vi "RT Driver VI.vi"(7 "Operation":T1, 11 "Device Reference in":T2 format="%.0x") -> (0 "Error Code":i32)   [LabVIEW 2019, in "FPGA Addon Engine.lvlib"]
uses:
  FPGA Addon Engine.lvlib
  <vilib>/rvi/interface/nirviCloseFPGA/nirviCloseFPGA.xnode
  <vilib>/FPGAPlugInAG/Dynamic/niLvFpga_Close_Dynamic.vi
  <vilib>/NI VeriStand/Custom Device API/Custom Device API.lvlib
  <vilib>/rvi/interface/nirviMethod/nirviMethod.xnode
  <vilib>/rvi/interface/nirviMethod/StockFPGA_InlinedMethodWaitForSingleIRQ.vi
  <vilib>/FPGAPlugInAG/Dynamic/niLvFpga_WaitOnIrq_Dynamic.vi
  <vilib>/FPGAPlugInAG/Dynamic/niLvFpga_AcknowledgeIrq_Dynamic.vi
  <vilib>/NI/NIVS Inline Async API/_VS Inline Async API/VS Inline Async API/VS Inline Async API.lvclass
  <vilib>/NI VeriStand/Custom Device Waveform API/Multiple Waveforms Write (DBL)/Multiple Waveforms Write (DBL).lvclass
  <vilib>/NI VeriStand/Custom Device Waveform API/Single Waveform Read (DBL)/Single Waveform Read (DBL).lvclass
  <vilib>/NI VeriStand/Custom Device API/Custom Device Item Ref.ctl
  <vilib>/NI VeriStand/Custom Device API/Hardware Interface Driver VI Operation.ctl
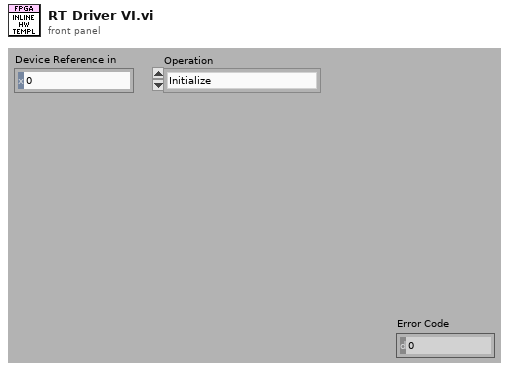
[diagram p1: front panel]
types:
  T1 = typedef "Custom Device API.lvlib/Hardware Interface Driver VI Operation.ctl" = enum16{"Initialize", "Start", "Read Data from HW", "Write Data to HW", "Close"}
  T2 = typedef "Custom Device API.lvlib/Custom Device Item Ref.ctl" = u64
  T3 = typedef "FPGA Addon Engine.lvlib/State Variables.ctl" = cluster{"FPGA Ref":refnum<k20>, "IncomingRegisters.Refs":T4[], "IncomingDMA.Refs":T7[], "OutgoingRegisters.Refs":T4[], "OutgoingDMA.Refs":T12[], "Compiled":T14}
  T4 = typedef "FPGA Addon Engine.lvlib/Register Settings.ctl" = cluster{"Data Type":T5, "U64":refnum<k20>, "U32":refnum<k20>, "U16":refnum<k20>, "U8":refnum<k20>, "I64":refnum<k20>, "I32":refnum<k20>, "I16":refnum<k20>, "I8":refnum<k20>, "SGL":refnum<k20>, "Bool":refnum<k20>, "Scalar Type":T6, "Index":i32, "Length":i32, "Analog PWM In":refnum<k20>, "Digital PWM In":refnum<k20>, "Digital PWM Out":refnum<k20>, "Analog PWM In Settings":refnum<k20>, "Digital PWM In Settings":refnum<k20>, "Sine Out":refnum<k20>, "FXP+/-24.5":refnum<k20>, "FXP+/-16.5":refnum<k20>, "FXP+/-32.8":refnum<k20>, "FXP+/-64.32":refnum<k20>, "FXP+/-16.7":refnum<k20>, "FXP+/-20.5":refnum<k20>, "FXP+/-27.5":refnum<k20>, "FXP+/-32.16":refnum<k20>, "FXP+16.3":refnum<k20>, "FXP+18.3":refnum<k20>, "Digital Static In":refnum<k20>, "Digital Static Out":refnum<k20>, "Digital Static In Settings":refnum<k20>, "Digital WSS Out":refnum<k20>, "Quad Encoder Settings":refnum<k20>, "Quad Encoder In":refnum<k20>}
  T5 = typedef "FPGA Addon Shared.lvlib/Data Type.ctl" = enum8{"<Null>", "I8", "I16", "I32", "I64", "U8", "U16", "U32", "U64", "SGL", "Boolean", "Analog PWM In Settings", "Analog PWM In", "Digital PWM In Settings", "Digital PWM In", "Digital PWM Out", "Sine Out", "FXP+/-24.5", "FXP+/-16.5", "FXP+/-32.8", "FXP+/-64.32", "FXP+/-16.7", "FXP+/-20.5", "FXP+/-27.5", "FXP+/-32.16", "FXP+16.3", "FXP+18.3", "Digital Static In", "Digital Static Out", "Digital Static In Settings", "Digital WSS Out", "Quad Encoder Settings", "Quad Encoder In", "Group"}
  T6 = typedef "FPGA Addon Shared.lvlib/Scalar Type.ctl" = enum16{"Standard", "Bitpacked"}
  T7 = typedef "FPGA Addon Engine.lvlib/DMA Input References.ctl" = cluster{"Addon Name":string, "Waveform Ref":refnum<class "Multiple Waveforms Write (DBL).lvclass">, "DMA Name":string, "DMA Settings":T8, "Refs":T11}
  T8 = typedef "FPGA Addon Shared.lvlib/DMA Settings.ctl" = cluster{"Number of Channels":u8, "Delacing Scheme":T9, "Update Rate":u32, "dt":dbl, "Mode":T10, "Number of Samples":u32, "DMA Host Buffer":u32}
  T9 = typedef "FPGA Addon Shared.lvlib/Delacing Scheme.ctl" = enum8{"Interleaved", "Bitpacked"}
  T10 = typedef "FPGA Addon Shared.lvlib/DMA Acquisition Mode.ctl" = enum8{"Continuous", "Triggered Finite"}
  T11 = typedef "FPGA Addon Engine.lvlib/DMA Input Refs.ctl" = cluster{"Data Type":T5, "DMA_SGL":refnum<k20>, "DMA_U64":refnum<k20>, "DMA_I64":refnum<k20>, "DMA_FXP+/-32.8":refnum<k20>, "DMA_FXP+/-64.32":refnum<k20>, "DMA_U32":refnum<k20>, "DMA_U16":refnum<k20>, "DMA_U8":refnum<k20>, "DMA_I32":refnum<k20>, "DMA_I16":refnum<k20>, "DMA_I8":refnum<k20>, "DMA_FXP+/-32.16":refnum<k20>}
  T12 = typedef "FPGA Addon Engine.lvlib/DMA Output References.ctl" = cluster{"Addon Name":string, "Waveforms":refnum<class "Single Waveform Read (DBL).lvclass">[], "DMA Name":string, "Refs":T13}
  T13 = typedef "FPGA Addon Engine.lvlib/DMA Output Refs.ctl" = cluster{"Data Type":T5, "DMA_SGL":refnum<k20>, "DMA_U64":refnum<k20>, "DMA_I64":refnum<k20>, "DMA_FXP+/-32.8":refnum<k20>, "DMA_FXP+/-64.32":refnum<k20>, "DMA_U32":refnum<k20>, "DMA_U16":refnum<k20>, "DMA_U8":refnum<k20>, "DMA_I32":refnum<k20>, "DMA_I16":refnum<k20>, "DMA_I8":refnum<k20>, "DMA_FXP+/-32.16":refnum<k20>}
  T14 = typedef "FPGA Addon Shared.lvlib/Compiled.Settings.ctl" = cluster{"Name":string, "IncomingRegisters.Settings":T15[], "IncomingRegisters.Refs":cluster{"Refs":T17[], "Values":dbl[]}, "OutgoingRegisters.Settings":T15[], "OutgoingRegisters.Refs":cluster{"Refs":T17[], "Values":dbl[]}, "Incoming.Size":i32, "Outgoing.Size":i32, "IncomingDMA.Settings":T19[], "OutgoingDMA.Settings":T19[], "FPGA.Settings":T21, "Target.Type":T22}
  T15 = typedef "FPGA Addon Shared.lvlib/Compiled.RegisterSettings.ctl" = cluster{"Scalar Type":T6, "Index":i32, "Length":i32, "Register":T16}
  T16 = typedef "FPGA Addon Shared.lvlib/Register Information.ctl" = cluster{"Name":string, "Data Type":T5, "Default Value":variant}
  T17 = typedef "Custom Device API.lvlib/Block Data Reference.ctl" = cluster{"Data Reference":T18, "Offset":u64, "Length":u64}
  T18 = typedef "Custom Device API.lvlib/Data Reference.ctl" = i32
  T19 = typedef "FPGA Addon Shared.lvlib/Compiled.DMASettings.ctl" = cluster{"Name":string, "Data Type":T5, "DMA.Settings":T8, "DMA.VSRefs":T20[]}
  T20 = typedef "Custom Device API.lvlib/Waveform Data Reference.ctl" = i32
  T21 = typedef "FPGA Addon Shared.lvlib/FPGA Settings.ctl" = cluster{"Bitfile path":path, "RIO Device Address":string, "Group":bool}
  T22 = typedef "Custom Device API.lvlib/Custom Device Target Type.ctl" = enum16{"PharLap", "VxWorks", "Windows", "Linux_32_ARM", "Linux_x64"}
  T23 = cluster{"Vars":T3, "Async?":bool, "Async":refnum<class "VS Inline Async API.lvclass">}
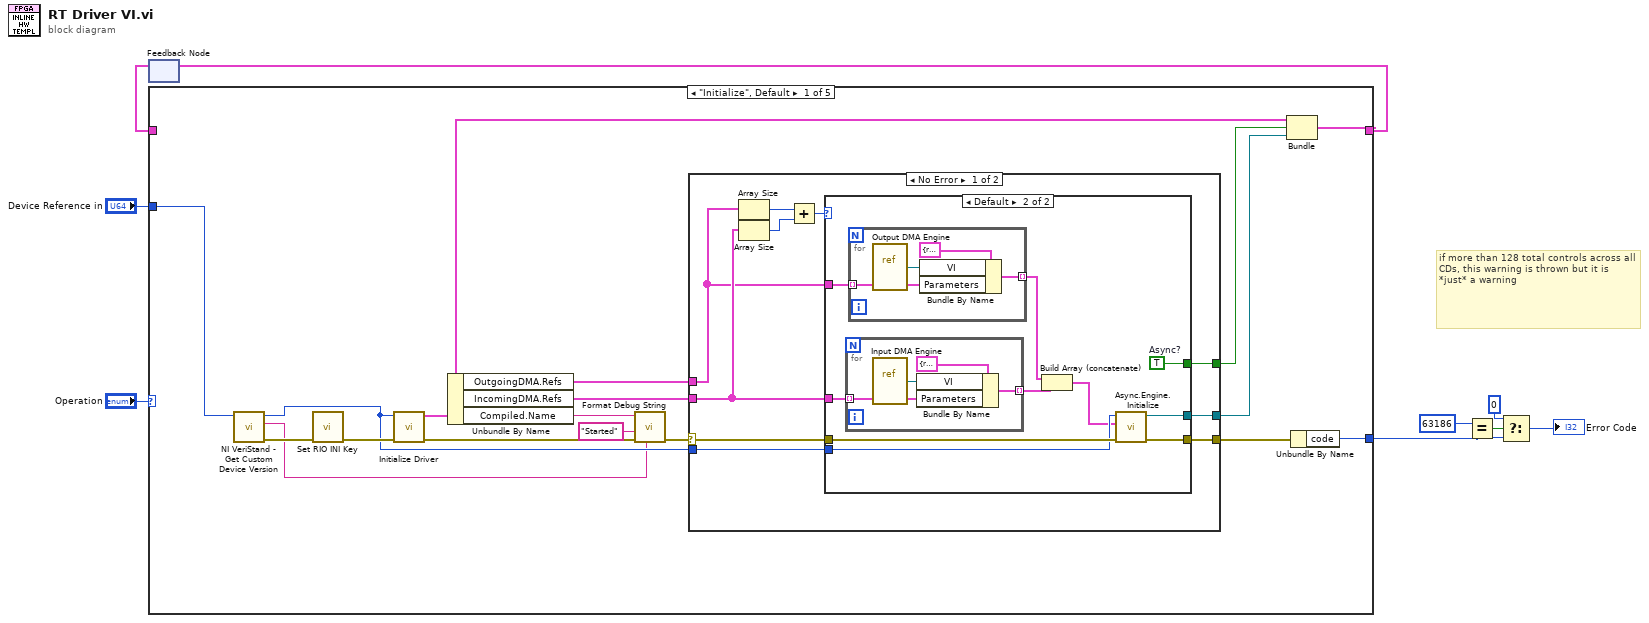
[diagram p0: block diagram]
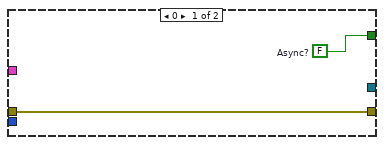
[diagram p2: hidden frame]
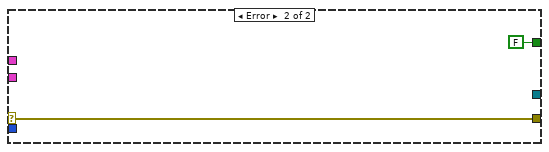
[diagram p3: hidden frame]
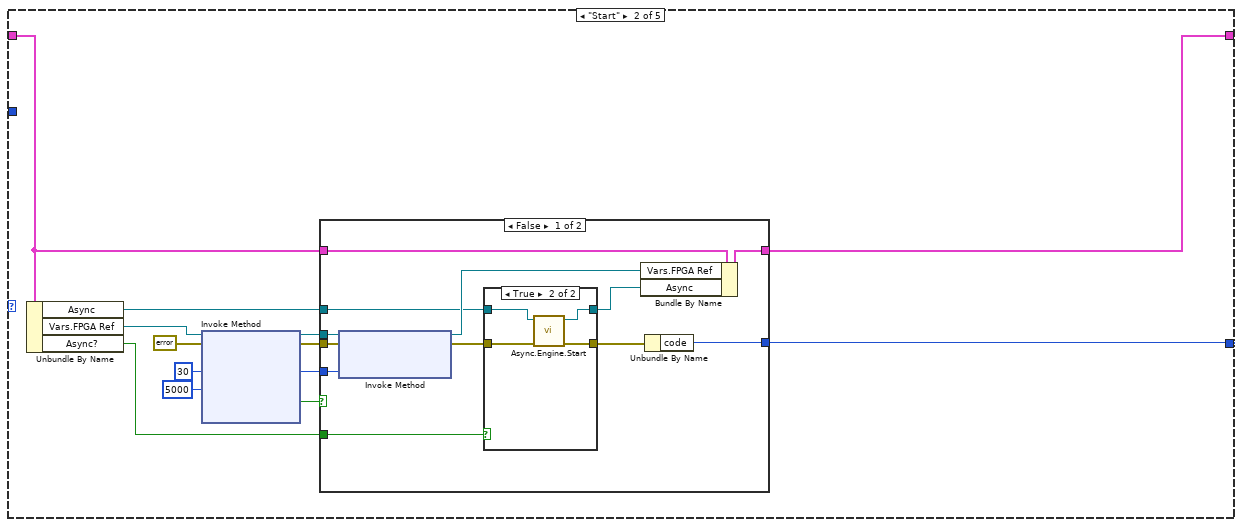
[diagram p4: hidden frame]
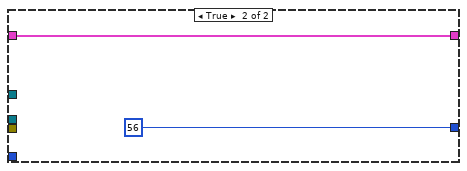
[diagram p6: hidden frame]
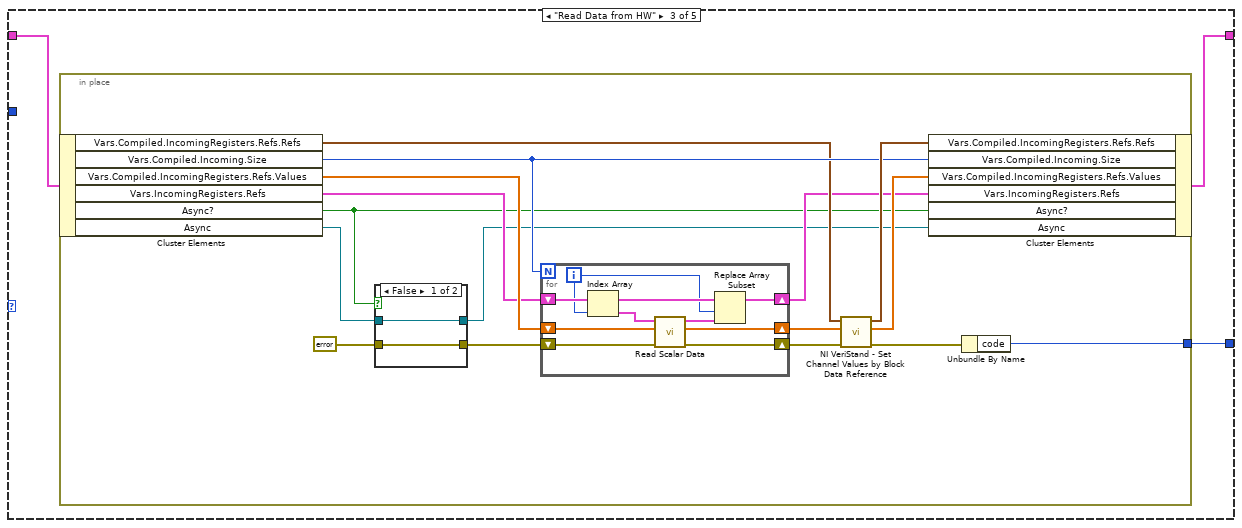
[diagram p7: hidden frame]
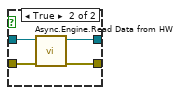
[diagram p8: hidden frame]
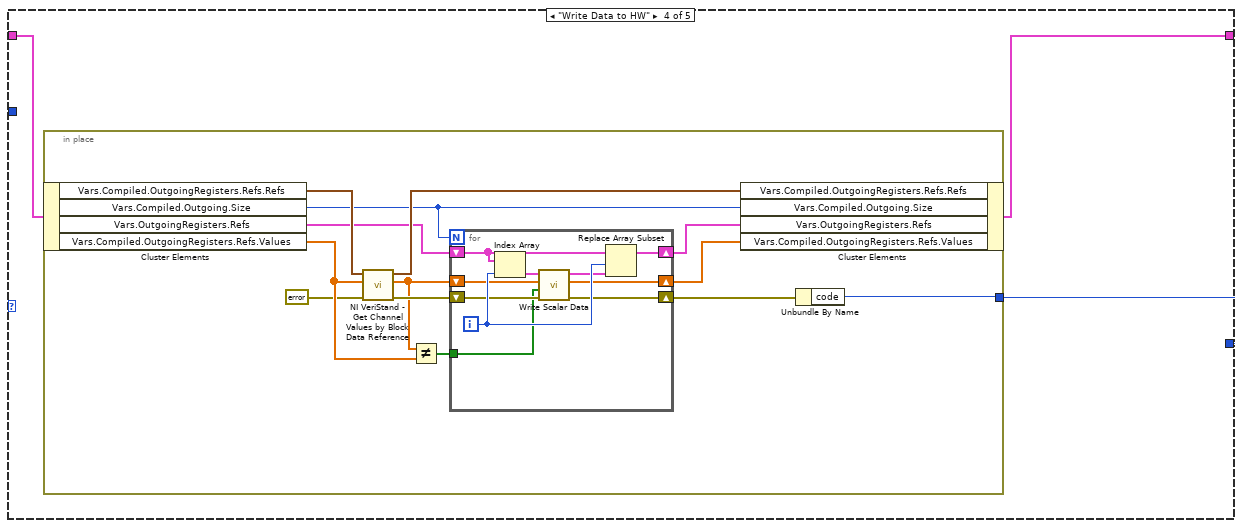
[diagram p9: hidden frame]
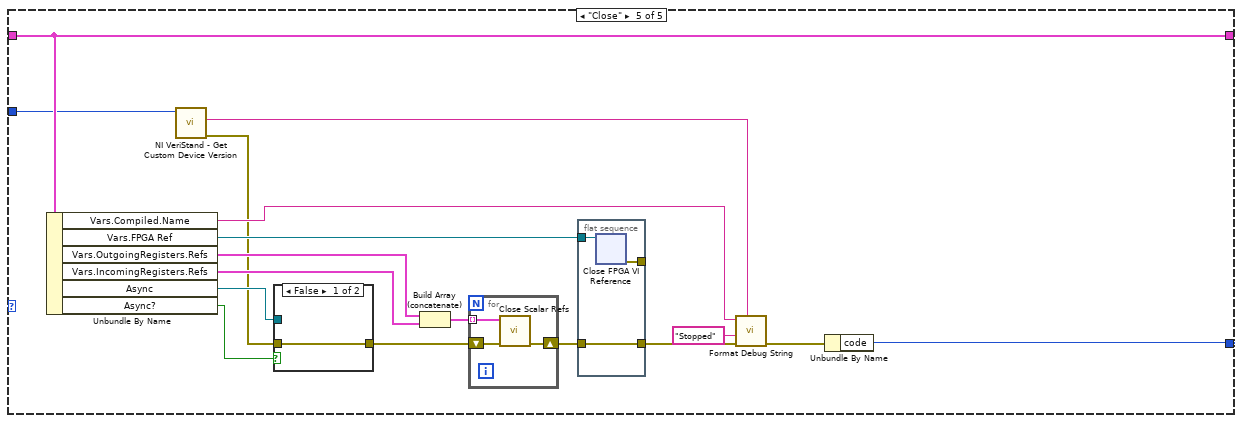
[diagram p10: hidden frame]
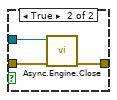
[diagram p11: hidden frame]
diagram:
  # "if more than 128 total controls across all CDs, this warning is thrown but it is *just* a warning"
  n1 = feedback #1() -> (w7:T23)  [unwired: 1 out]
  n2 = case shown="\"Initialize\", Default" "Operation" {
    tunnel: [w26 w68 w93 w126 w165] -> w8
    tunnel: w7 -> [_ w69 w91 w127 w165]
    tunnel: "Device Reference in" -> [w16 _ _ _ w157]
    tunnel: [w25 w70 w92 w125 w167] -> w4
    frame "Initialize", Default {
      n3 = call <vilib>:"NI VeriStand - Get Custom Device Version.vi"("Device Ref in"=w16) -> ("error out"=w17:errorcluster, "Value"=w13:string, "Device Ref out"=w15:T2)  [unwired: 8 in]
      n4 = call "Set RIO INI Key.vi"("error in (no error)"=w17) -> ("error out"=w24:errorcluster)  [unwired: 10 in]
      n5 = call "Initialize Driver.vi"("error in (no error)"=w24, "Section Ref in"=w15) -> ("error out"=w14:errorcluster, "Vars"=w18:T3)  [unwired: 8 in]
      n6 = Unbundle By Name(w18) -> ("OutgoingDMA.Refs"=w20:T12[], "IncomingDMA.Refs"=w21:T7[], "Compiled.Name"=w12:string)
      n7 = call "Format Debug String.vi"("Version"=w13, "error in (no error)"=w14, "State"="Started" ("string"), "Name"=w12) -> ("error out"=w10:errorcluster)  [unwired: 7 in]
      n8 = case shown="No Error" w10 {
        selector: w10 -> [w27 w58]
        tunnel: [w36 w58] -> w23
        tunnel: [w35 _] -> w22
        tunnel: w21 -> [w34 _]
        tunnel: w20 -> [w33 _]
        tunnel: [w29 FALSE ("Async?")] -> w19
        tunnel: w15 -> [w28 _]
        frame No Error {
          n9 = Array Size(array=w33) -> (size(s)=w32:i32)
          n10 = Array Size(array=w34) -> (size(s)=w31:i32)
          n11 = Add(x=w32, y=w31) -> (x+y=w30:i32)
          n12 = case shown="Default" w30 {
            tunnel: w27 -> [w38 w45]
            tunnel: [w38 w44] -> w36
            tunnel: [_ w43] -> w35
            tunnel: w34 -> [_ w41]
            tunnel: w33 -> [_ w48]
            tunnel: [w37 w46] -> w29
            tunnel: w28 -> [_ w42]
            frame 0 {
              w37 = FALSE  # Async?
            }
            frame Default {
              w46 = TRUE  # Async?
              n13 = for {
                tunnel: w41 -> [w49] mode=indexing
                tunnel: [w51] -> w40 mode=indexing
                n14 = vi-ref "Input DMA Engine.vi"() -> (w50:refnum<vi>)
                n15 = Bundle By Name(cluster=cluster{"VI":refnum<vi>, "Parameters":variant} {"VI"=refnum, "Parameters"=variant} ("Process"), "VI"=w50, "Parameters"=w49) -> (w51:cluster{"VI":refnum<vi>, "Parameters":variant})
              }
              n16 = for {
                tunnel: w48 -> [w55] mode=indexing
                tunnel: [w54] -> w47 mode=indexing
                n17 = vi-ref "Output DMA Engine.vi"() -> (w53:refnum<vi>)
                n18 = Bundle By Name(cluster=cluster{"VI":refnum<vi>, "Parameters":variant} {"VI"=refnum, "Parameters"=variant} ("Process"), "VI"=w53, "Parameters"=w55) -> (w54:cluster{"VI":refnum<vi>, "Parameters":variant})
              }
              n19 = Build Array (concatenate)(w47, w40) -> (w39:cluster{"VI":refnum<vi>, "Parameters":variant}[])
              n20 = call <vilib>:"Async.Engine.Initialize.vi"("error in (no error)"=w45, "Processes"=w39, "Custom Device Ref"=w42) -> ("error out"=w44:errorcluster, "Async"=w43:refnum<class "VS Inline Async API.lvclass">)  [unwired: 7 in]
            }
          }
        }
        frame Error {
        }
      }
      n21 = Bundle("Vars"=w18, "Async?"=w19, "Async"=w22) -> (w26:T23)  [unwired: 1 out]
      n22 = Unbundle By Name(w23) -> ("code"=w25:i32)
    }
    frame "Start" {
      w64 = 30 ("IRQ Number(s)")
      n23 = Unbundle By Name(w69) -> ("Async"=w60:refnum<class "VS Inline Async API.lvclass">, "Vars.FPGA Ref"=w67:refnum<k20>, "Async?"=w62:bool)
      n24 = xnode "Invoke Method"("FPGA VI Reference In"=w67, "error in"=errorcluster {"status"=FALSE, "code"=0, "source"=""}, "IRQ Number(s)"=w64, "Timeout (ms)"=5000) -> ("FPGA VI Reference Out"=w66:refnum<k20>, "error out"=w65:errorcluster, "Timed Out"=w61:bool)  [unwired: 1 out]
      n25 = case shown="False" w61 {
        tunnel: [w82 56 ("code")] -> w70
        tunnel: w69 -> [w81 w90]
        tunnel: [w80 w90] -> w68
        tunnel: w66 -> [w79 _]
        tunnel: w65 -> [w78 _]
        tunnel: w64 -> [w77 _]
        tunnel: w62 -> [w74 _]
        tunnel: w60 -> [w73 _]
        frame False {
          n26 = xnode "Invoke Method"("FPGA VI Reference In"=w79, "error in"=w78, "IRQ Number(s)"=w77) -> ("FPGA VI Reference Out"=w76:refnum<k20>, "error out"=w71:errorcluster)
          n27 = case shown="True" w74 {
            tunnel: w71 -> [w84 w88]
            tunnel: [w84 w87] -> w75
            tunnel: w73 -> [w83 w86]
            tunnel: [w83 w85] -> w72
            frame False {
            }
            frame True {
              n28 = call <vilib>:"Async.Engine.Start.vi"("error in (no error)"=w88, "VS Inline Async API in"=w86) -> ("error out"=w87:errorcluster, "VS Inline Async API out"=w85:refnum<class "VS Inline Async API.lvclass">)  [unwired: 8 in]
            }
          }
          n29 = Bundle By Name(cluster=w81, "Vars.FPGA Ref"=w76, "Async"=w72) -> (w80:T23)
          n30 = Unbundle By Name(w75) -> ("code"=w82:i32)
        }
        frame True {
        }
      }
    }
    frame "Read Data from HW" {
      n31 = in-place {
        in-place-border: [w99] -> w92
        n32 = in-place-cluster #2(w91) -> ("Vars.Compiled.IncomingRegisters.Refs.Refs"=w103:T17[], "Vars.Compiled.Incoming.Size"=w105:i32, "Vars.Compiled.IncomingRegisters.Refs.Values"=w109:dbl[], "Vars.IncomingRegisters.Refs"=w102:T4[], "Async?"=w95:bool, "Async"=w97:refnum<class "VS Inline Async API.lvclass">)
        n33 = case shown="False" w95 {
          tunnel: w97 -> [w111 w115]
          tunnel: [w110 w114] -> w98
          tunnel: [w111 w113] -> w96
          tunnel: errorcluster {"status"=FALSE, "code"=0, "source"=""} ("error in") -> [w110 w112]
          frame False {
          }
          frame True {
            n34 = call <vilib>:"Async.Engine.Read Data from HW.vi"("error in"=w112, "Async in"=w115) -> ("error out"=w114:errorcluster, "Async out"=w113:refnum<class "VS Inline Async API.lvclass">)  [unwired: 8 in]
          }
        }
        n35 = for {
          N: w105 -> [_]
          shift-right: [w116] -> w106
          shift-left: w109 -> [w117]
          shift-right: [w124] -> w101
          shift-left: w102 -> [w123]
          shift-right: [w121] -> w104
          shift-left: w98 -> [w122]
          i -> [w118]
          n36 = Index Array(array=w123, index=w118) -> (element=w119:T4)
          n37 = call "Read Scalar Data.vi"("error in (no error)"=w122, "Values"=w117, "Cluster"=w119) -> ("error out"=w121:errorcluster, "Values"=w116:dbl[], "Cluster"=w120:T4)  [unwired: 6 in]
          n38 = Replace Array Subset(array=w123, new element=w120, index=w118) -> (w124:T4[])
        }
        n39 = call <vilib>:"NI VeriStand - Set Channel Values by Block Data Reference.vi"("error in (no error)"=w104, "Values Array in"=w106, "Block Data Ref"=w103) -> ("error out"=w100:errorcluster, "Values Array out"=w107:dbl[], "Block Data Ref dup"=w108:T17[])  [unwired: 6 in]
        n40 = in-place-cluster #2("Vars.Compiled.IncomingRegisters.Refs.Refs"=w108, "Vars.Compiled.Incoming.Size"=w105, "Vars.Compiled.IncomingRegisters.Refs.Values"=w107, "Vars.IncomingRegisters.Refs"=w101, "Async?"=w95, "Async"=w96) -> (w93:T23)
        n41 = Unbundle By Name(w100) -> ("code"=w99:i32)
      }
    }
    frame "Write Data to HW" {
      n42 = in-place {
        in-place-border: [w132] -> w125
        n43 = in-place-cluster #3(w127) -> ("Vars.Compiled.OutgoingRegisters.Refs.Refs"=w140:T17[], "Vars.Compiled.Outgoing.Size"=w134:i32, "Vars.OutgoingRegisters.Refs"=w138:T4[], "Vars.Compiled.OutgoingRegisters.Refs.Values"=w130:dbl[])
        n44 = call <vilib>:"NI VeriStand - Get Channel Values by Block Data Reference.vi"("error in (no error)"=errorcluster {"status"=FALSE, "code"=0, "source"=""} ("error in"), "Values Array in"=w130, "Block Data Ref"=w140) -> ("error out"=w135:errorcluster, "Values Array out"=w131:dbl[], "Block Data Ref dup"=w139:T17[])  [unwired: 6 in]
        n45 = Not Equal?(x=w131, y=w130) -> (x != y?=w129:bool[])
        n46 = for {
          N: w134 -> [_]
          shift-right: [w142] -> w136
          shift-left: w131 -> [w143]
          shift-right: [w150] -> w137
          shift-left: w138 -> [w149]
          shift-right: [w145] -> w133
          shift-left: w135 -> [w146]
          tunnel: w129 -> [w141]
          i -> [w148]
          n47 = Index Array(array=w149, index=w148) -> (element=w144:T4)
          n48 = call "Write Scalar Data.vi"("error in (no error)"=w146, "Changed?"=w141, "Values"=w143, "Cluster"=w144) -> ("error out"=w145:errorcluster, "Values"=w142:dbl[], "Cluster"=w147:T4)  [unwired: 5 in]
          n49 = Replace Array Subset(array=w149, new element=w147, index=w148) -> (w150:T4[])
        }
        n50 = in-place-cluster #3("Vars.Compiled.OutgoingRegisters.Refs.Refs"=w139, "Vars.Compiled.Outgoing.Size"=w134, "Vars.OutgoingRegisters.Refs"=w137, "Vars.Compiled.OutgoingRegisters.Refs.Values"=w136) -> (w126:T23)
        n51 = Unbundle By Name(w133) -> ("code"=w132:i32)
      }
    }
    frame "Close" {
      n52 = Unbundle By Name(w165) -> ("Vars.Compiled.Name"=w152:string, "Vars.FPGA Ref"=w161:refnum<k20>, "Vars.OutgoingRegisters.Refs"=w164:T4[], "Vars.IncomingRegisters.Refs"=w163:T4[], "Async"=w158:refnum<class "VS Inline Async API.lvclass">, "Async?"=w160:bool)
      n53 = call <vilib>:"NI VeriStand - Get Custom Device Version.vi"("Device Ref in"=w157) -> ("error out"=w151:errorcluster, "Value"=w153:string)  [unwired: 8 in, 1 out]
      n54 = case shown="False" w160 {
        tunnel: [w168 w171] -> w162
        tunnel: w158 -> [_ w170]
        tunnel: w151 -> [w168 w169]
        frame False {
        }
        frame True {
          n55 = call <vilib>:"Async.Engine.Close.vi"("error in (no error)"=w169, "Async in"=w170) -> ("error out"=w171:errorcluster)  [unwired: 8 in, 1 out]
        }
      }
      n56 = Build Array (concatenate)(w164, w163) -> (w166:T4[])
      n57 = for {
        tunnel: w166 -> [w175] mode=indexing
        shift-right: [w176] -> w159
        shift-left: w162 -> [w177]
        n58 = call "Close Scalar Refs.vi"("error in (no error)"=w177, "Cluster"=w175) -> ("error out"=w176:errorcluster)  [unwired: 9 in]
      }
      n59 = flat-sequence {
        tunnel: w159 -> [w174]
        tunnel: w161 -> [w173]
        tunnel: [w174] -> w154
        tunnel: [w172] -> _
        frame #0 {
          n60 = xnode "Close FPGA VI Reference"("FPGA VI Reference In"=w173) -> ("error out"=w172:errorcluster)  [unwired: 1 in]
        }
      }
      n61 = call "Format Debug String.vi"("Version"=w153, "error in (no error)"=w154, "State"="Stopped" ("string"), "Name"=w152) -> ("error out"=w155:errorcluster)  [unwired: 7 in]
      n62 = Unbundle By Name(w155) -> ("code"=w167:i32)
    }
  }
  n63 = feedback-in #1(w8) -> ()
  n64 = Equal?(x=63186, y=w4) -> (x = y?=w5:bool)
  n65 = Select(t=0, s=w5, f=w4) -> (s? t:f=→"Error Code":i32)
